vi "check for perc change.vi"(1 "Numeric":dbl format="%#_13g") -> (0 "Numeric 2":dbl format="%#_13g")   [LabVIEW 2015]
panel:
  in  "y":dbl=0.1 format="%#_13g"
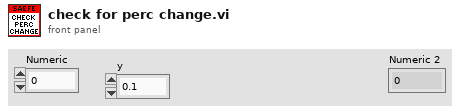
[diagram p1: front panel]
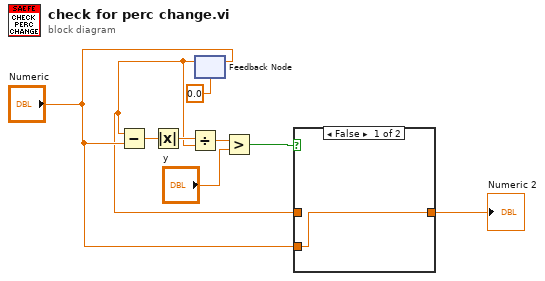
[diagram p0: block diagram]
diagram:
  n1 = feedback-in #1("Numeric") -> ()
  n2 = feedback #1(0.0) -> (w1:dbl)
  n3 = Subtract(x=w1, y="Numeric") -> (x-y=w8:dbl)
  n4 = Absolute Value(x=w8) -> (abs(x)=w7:dbl)
  n5 = Divide(x=w7, y=w1) -> (x/y=w6:dbl)
  n6 = Greater?(x=w6, y="y") -> (0:w4:bool)
  n7 = case shown="False" w4 {
    tunnel: "Numeric" -> [w10 _]
    tunnel: [w10 w11] -> w2
    tunnel: w1 -> [_ w11]
    frame False {
    }
    frame True {
    }
  }
  "Numeric 2" <- w2
